vi "GT Arc ZXC.vi"(0 "cardNum":i16, 1 "zCenter":dbl, 2 "circleDir":i16, 3 "synAcc":dbl, 5 "crd":i16, 7 "z":i32, 9 "x":i32, 10 "fifo":i16, 11 "error in (no error)":errorcluster caption="错误输入（无错误）", 12 "xCenter":dbl, 13 "synVel":dbl, 14 "velEnd":dbl) -> (4 "cardNum":i16, 15 "error out":errorcluster caption="错误输出")   [LabVIEW 2020, in "gts.lvlib"]
doc: "GT_API GT_ArcZXC(short cardNum,short crd,long z,long x,double zCenter,double xCenter,short circleDir,double synVel,double synAcc,double velEnd=0,short fifo=0);"
uses:
  gts.lvlib
  dll/32bit/multi_card/gts.dll
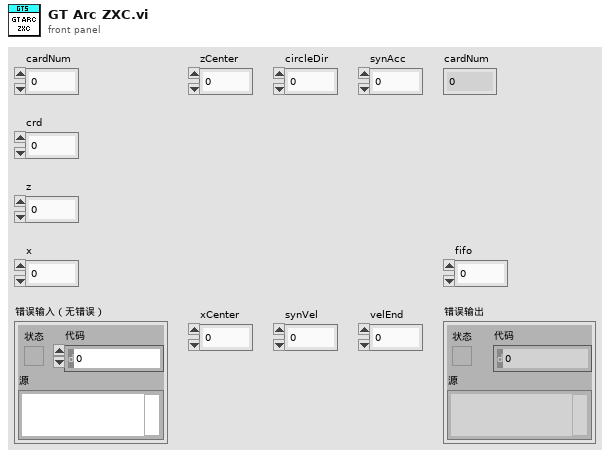
[diagram p1: front panel]
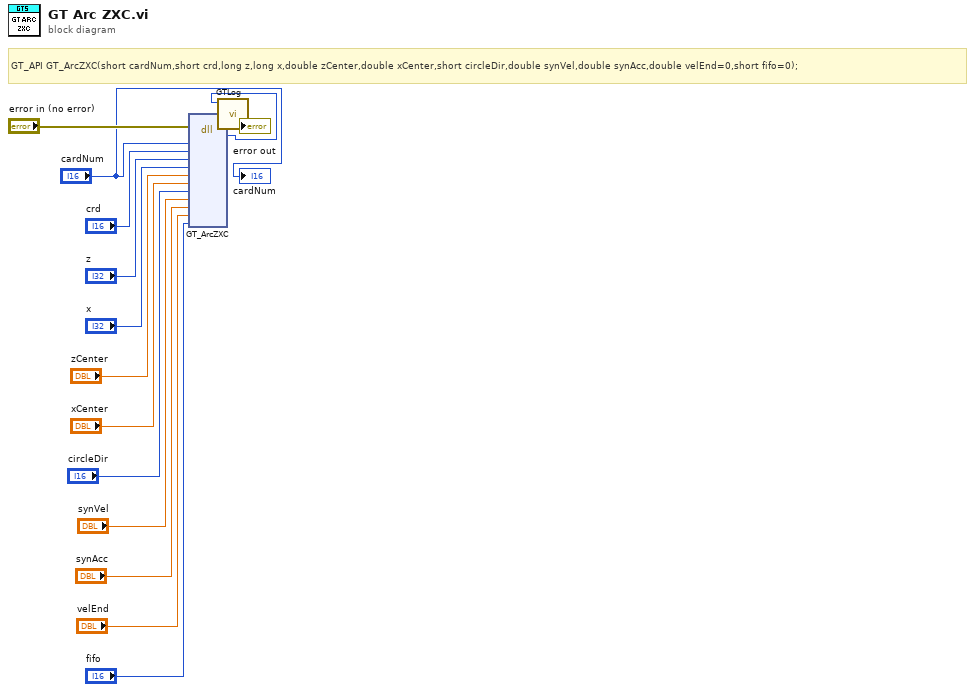
[diagram p0: block diagram]
diagram:
  # "GT_API GT_ArcZXC(short cardNum,short crd,long z,long x,double zCenter,double xCenter,short circleDir,double synVel,double synAcc,double velEnd=0,short fifo=0);"
  n1 = dll-call lib="D:/Git/GoogolCard/dll/32bit/multi_card/gts.dll" fn="GT_ArcZXC"(error in="error in (no error)", "cardNum"="cardNum", "crd"="crd", "z"="z", "x"="x", "zCenter"="zCenter", "xCenter"="xCenter", "circleDir"="circleDir", "synVel"="synVel", "synAcc"="synAcc", "velEnd"="velEnd", "fifo"="fifo") -> (error out=w4:errorcluster, w2:i16)  [unwired: 13 in, 1 out]
  n2 = call "GTLog.vi"("error in (no error)"=w4, "Numeric"=w2) -> ("error out"=→"error out":errorcluster)  [unwired: 9 in]
  "cardNum" <- "cardNum"
